vi "Set Line Color.vi"(9 "data row index":i32, 10 "line color":u32(colorbox)=16711680, 11 "draw options in":T1={"Background Color"=16777215, "Grid Color"=13816530, "Angle Units"=enum."Radians", "Draw Solid Background"=TRUE, "Draw Grid"=TRUE, "Grid Spacing"=1.0, "AutoScale"=TRUE, "Fit to Radius"=1.0, "data row options"=[]}) -> (3 "draw options out":T1={"Background Color"=16777215, "Grid Color"=13816530, "Angle Units"=enum."Radians", "Draw Solid Background"=TRUE, "Draw Grid"=TRUE, "Grid Spacing"=1.0, "AutoScale"=TRUE, "Fit to Radius"=1.0, "data row options"=[]})   [LabVIEW 2017, in "NI_Robotics_2D Rangefinder Picture.lvlib"]
uses:
  <vilib>/robotics/Controls/2D Rangefinder/2D Rangefinder Picture/NI_Robotics_2D Rangefinder Picture.lvlib
  <vilib>/robotics/Controls/2D Rangefinder/2D Rangefinder Picture/Draw Options.ctl
  <vilib>/robotics/Controls/Utilities/Angle Units.ctl
  <vilib>/robotics/Controls/2D Rangefinder/2D Rangefinder Picture/Data Row Options.ctl
  <vilib>/robotics/Controls/Utilities/NI_Robotics_Control Utilities.lvlib
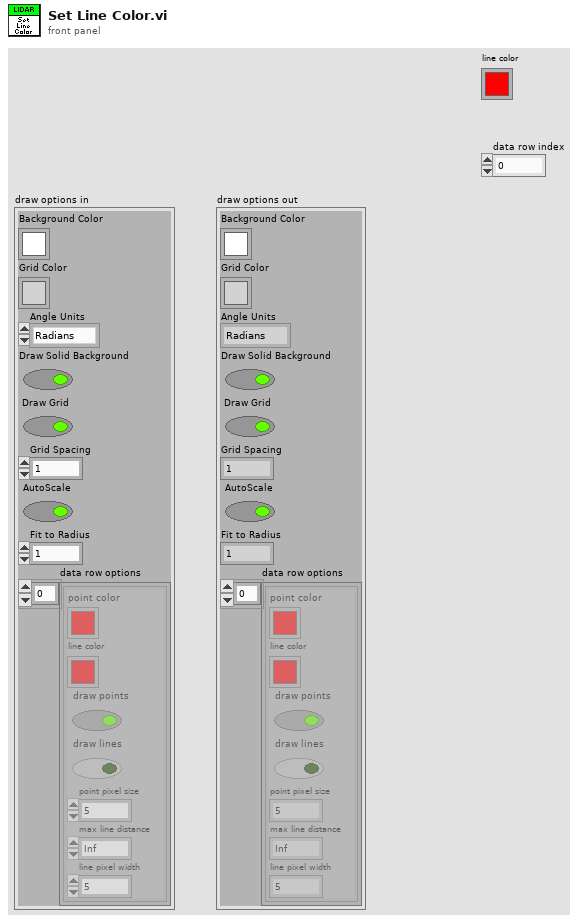
[diagram p1: front panel]
types:
  T1 = typedef "NI_Robotics_2D Rangefinder Picture.lvlib/Draw Options.ctl" = cluster{"Background Color":u32, "Grid Color":u32, "Angle Units":T2, "Draw Solid Background":bool, "Draw Grid":bool, "Grid Spacing":dbl, "AutoScale":bool, "Fit to Radius":dbl, "data row options":T3[]}
  T2 = typedef "NI_Robotics_Control Utilities.lvlib/Angle Units.ctl" = enum16{"Radians", "Degrees"}
  T3 = typedef "NI_Robotics_2D Rangefinder Picture.lvlib/Data Row Options.ctl" = cluster{"point color":u32, "line color":u32, "draw points":bool, "draw lines":bool, "point pixel size":u16, "max line distance":dbl, "line pixel width":u16}
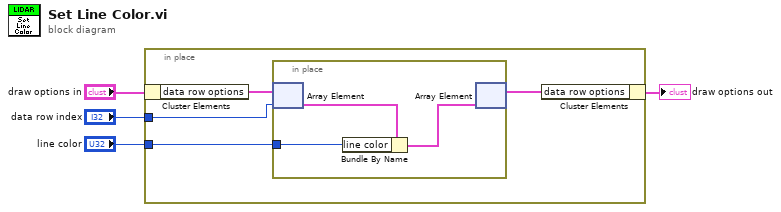
[diagram p0: block diagram]
diagram:
  n1 = in-place {
    in-place-border: "data row index" -> [w6]
    in-place-border: "line color" -> [w5]
    n2 = in-place-cluster #1("draw options in") -> ("data row options"=w8:T3[])
    n3 = in-place {
      in-place-border: w5 -> [w9]
      n4 = in-place-array #2(w8, w6) -> (w11:T3)
      n5 = Bundle By Name(cluster=w11, "line color"=w9) -> (w10:T3)
      n6 = in-place-array #2(w10) -> (w7:T3[])  [unwired: 1 out]
    }
    n7 = in-place-cluster #1("data row options"=w7) -> (→"draw options out":T1)
  }
